vi "Open Interface.vi"(6 "read_timeout (1000)":i32=1000, 8 "error in (no error)":errorcluster, 9 "capture_size (65536)":i32=65536, 10 "promiscuous mode (T)":bool=TRUE, 11 "adapter (0)":i32) -> (0 "error out":errorcluster, 3 "pcap reference":u64)   [LabVIEW 2025, in "Automotive Ethernet Bus Monitor UI.lvlib" / "lvwpcap.lvlib"]
doc: "Opens the interface to a specified ethernet adapter."
uses:
  lvwpcap.lvlib
  lvwpcap.dll
panel:
  in  "pcap (dummy)":u32
  # "Select Help»Show Context Help and move the cursor over the VI icon to display help for this VI."
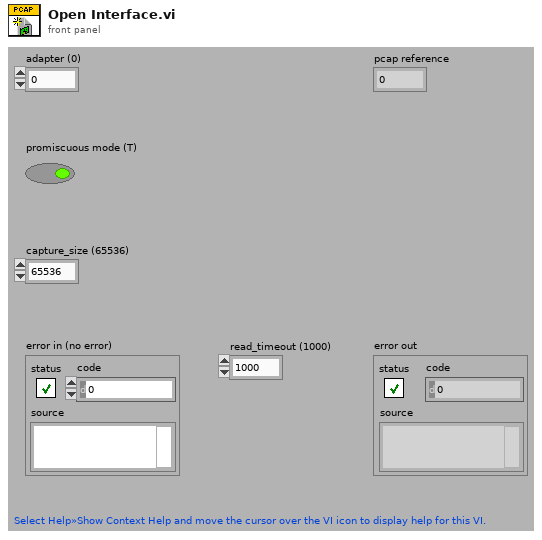
[diagram p1: front panel]
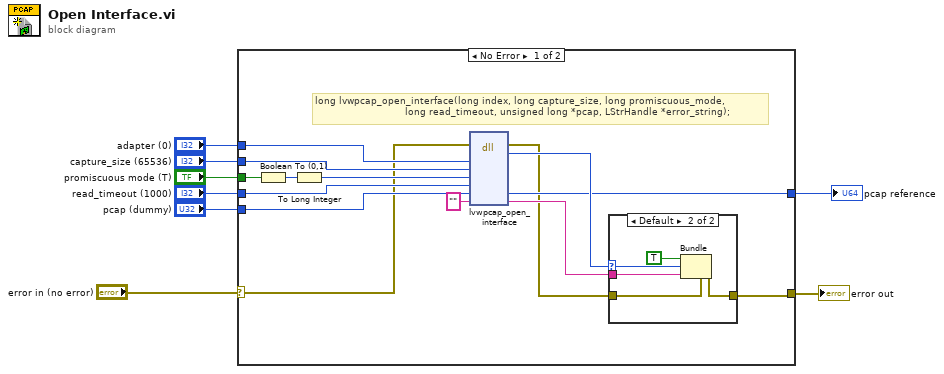
[diagram p0: block diagram]
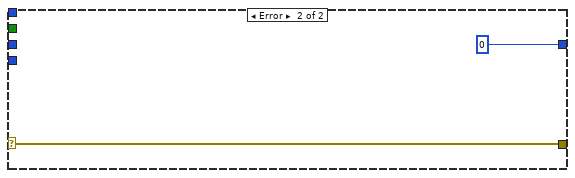
[diagram p3: hidden frame]
diagram:
  n1 = case shown="No Error" "error in (no error)" {
    selector: "error in (no error)" -> [w11 w30]
    tunnel: [w18 w30] -> w7
    tunnel: "pcap (dummy)" -> [w17 _]
    tunnel: "read_timeout (1000)" -> [w16 _]
    tunnel: "promiscuous mode (T)" -> [w15 _]
    tunnel: "capture_size (65536)" -> [w14 _]
    tunnel: "adapter (0)" -> [w13 _]
    tunnel: [w12 u64 0 ("pcap")] -> w1
    frame No Error {
      # "long lvwpcap_open_interface(long index, long capture_size, long promiscuous_mode,\n                              long read_timeout, unsigned long *pcap, LStrHandle *error_string);"
      n2 = Boolean To (0,1)(Boolean=w15) -> (0, 1=w20:i16)
      n3 = To Long Integer(number=w20) -> (32bit integer=w19:i32)
      n4 = dll-call lib="lvwpcap.dll" fn="lvwpcap_open_interface"(error in=w11, "index"=w13, "capture_size"=w14, "promiscuous_mode"=w19, "read_timeout"=w16, "pcap"=w17, "error_string"="") -> (error out=w10:errorcluster, "return type"=w22:i32, "pcap"=w12:u64, "error_string"=w21:string)  [unwired: 6 in, 1 out]
      n5 = case shown="Default" w22 {
        selector: w22 -> [_ w27]
        tunnel: w21 -> [_ w26]
        tunnel: w10 -> [w23 w28]
        tunnel: [w23 w24] -> w18
        frame 0 {
        }
        frame Default {
          n6 = Bundle(cluster=w28, "status"=TRUE, "code"=w27, "source"=w26) -> (w24:errorcluster)
        }
      }
    }
    frame Error {
    }
  }
  "error out" <- w7
  "pcap reference" <- w1
